vi "hw9p6_hickey.vi"() -> ()   [LabVIEW 2014]
panel:
  out "Output":dbl caption="Output: Deg F"
  in  "Input":dbl caption="Input: Deg C"
  in  "Enum":enum16{"F to C", "C to F"}(ring)
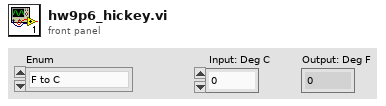
[diagram p1: front panel]
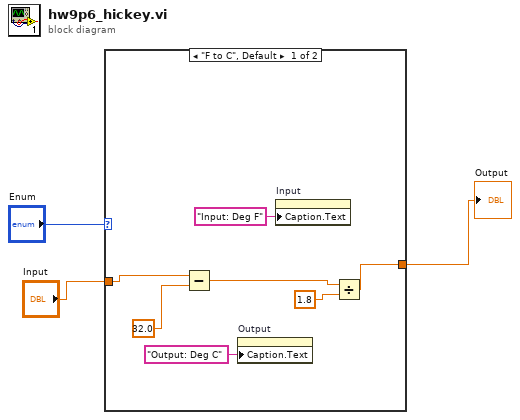
[diagram p0: block diagram]
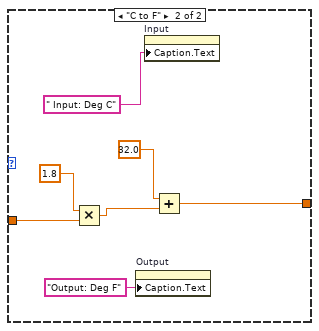
[diagram p2: hidden frame]
diagram:
  n1 = case shown="\"F to C\", Default" "Enum" {
    tunnel: "Input" -> [w7 w17]
    tunnel: [w9 w13] -> w1
    frame "F to C", Default {
      n2 = Subtract(x=w7, y=32.0) -> (x-y=w10:dbl)
      n3 = property on="Output" class="DigNum (strict)"("Caption.Text"="Output: Deg C") -> ()  [unwired: 2 in, 2 out]
      n4 = property on="Input" class="DigNum (strict)"("Caption.Text"="Input: Deg F") -> ()  [unwired: 2 in, 2 out]
      n5 = Divide(x=w10, y=1.8) -> (x/y=w9:dbl)
    }
    frame "C to F" {
      n6 = Multiply(x=1.8, y=w17) -> (x*y=w15:dbl)
      n7 = property on="Output" class="DigNum (strict)"("Caption.Text"="Output: Deg F") -> ()  [unwired: 2 in, 2 out]
      n8 = property on="Input" class="DigNum (strict)"("Caption.Text"=" Input: Deg C") -> ()  [unwired: 2 in, 2 out]
      n9 = Add(x=32.0, y=w15) -> (x+y=w13:dbl)
    }
  }
  "Output" <- w1
